vi "MPU_Stick_Write_General_Parameter.vi"(0 "ADCP in":refnum<class "ADCP.lvclass">, 5 "Parameter Name":string, 7 "Parameter Value":string, 11 "error out":errorcluster) -> (4 "ADCP out":refnum<class "ADCP.lvclass">, 15 "error out":errorcluster)   [LabVIEW 2017]
uses:
  Classes/ADCP.lvclass
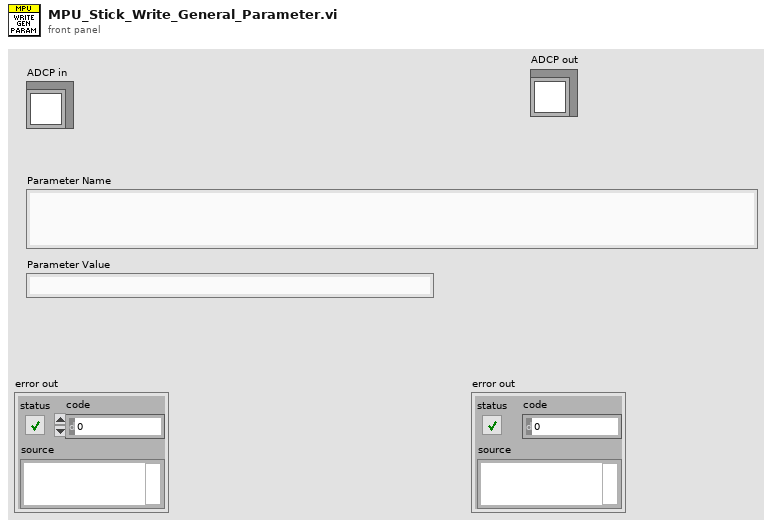
[diagram p1: front panel]
types:
  T1 = typedef "ADCP.lvclass/ADCP_Packet_Info.ctl" = cluster{"Priority":enum16{"LOW", "HIGH"}, "Type":enum16{"Data", "Connection Management", "Remote Request", "Error and status", "INVALID"}, "Node ID":i32, "Frame ID":i32, "Checksum valid ?":bool, "Current time (ms)":u32}
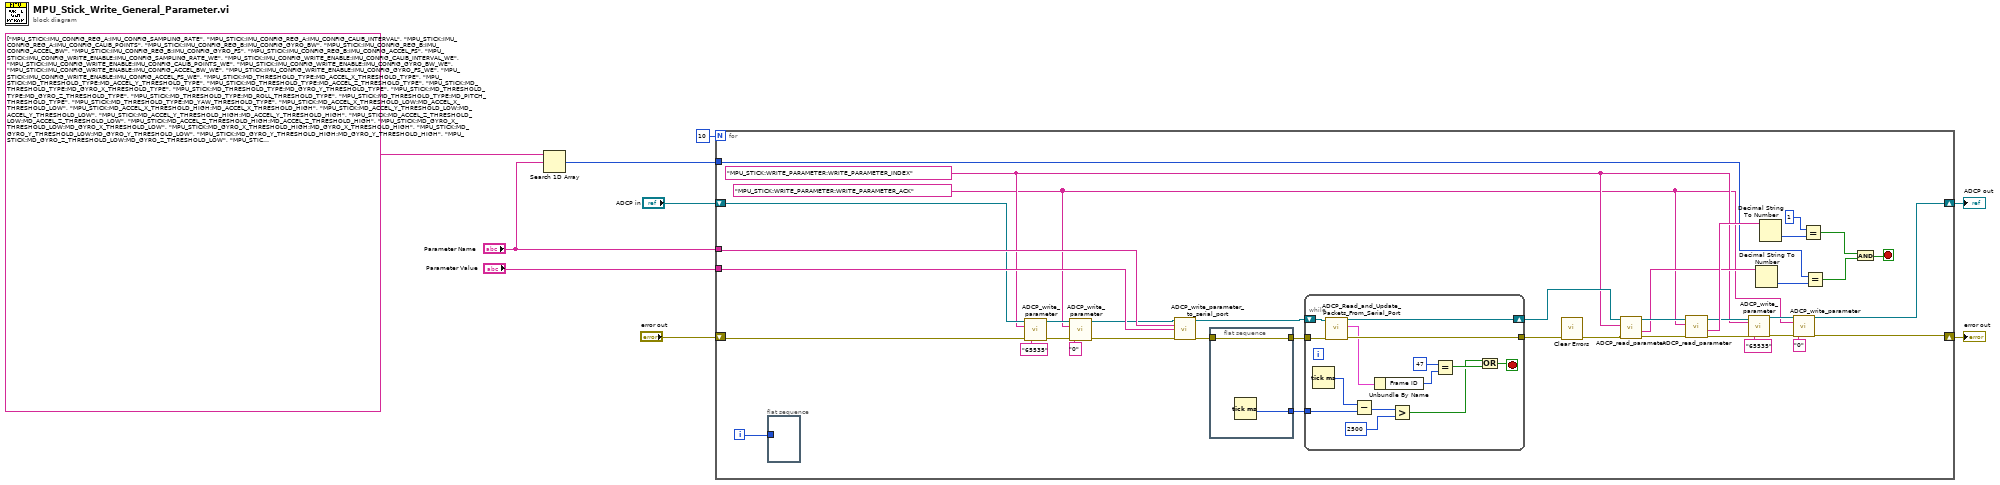
[diagram p0: block diagram]
diagram:
  n1 = Search 1D Array(1D array=string[] ["MPU_STICK:IMU_CONFIG_REG_A:IMU_CONFIG_SAMPLING_RATE", "MPU_STICK:IMU_CONFIG_REG_A:IMU_CONFIG_CALIB_INTERVAL", "MPU_STICK:IMU_CONFIG_REG_A:IMU_CONFIG_CALIB_POINTS", "MPU_STICK:IMU_CONFIG_REG_B:IMU_CONFIG_GYRO_BW", "MPU_STICK:IMU_CONFIG_REG_B:IMU_CONFIG_ACCEL_BW", "MPU_STICK:IMU_CONFIG_REG_B:IMU_CONFIG_GYRO_FS", "MPU_STICK:IMU_CONFIG_REG_B:IMU_CONFIG_ACCEL_FS", "MPU_STICK:IMU_CONFIG_WRITE_ENABLE:IMU_CONFIG_SAMPLING_RATE_WE", "MPU_STICK:IMU_CONFIG_WRITE_ENABLE:IMU_CONFIG_CALIB_INTERVAL_WE", "MPU_STICK:IMU_CONFIG_WRITE_ENABLE:IMU_CONFIG_CALIB_POINTS_WE", "MPU_STICK:IMU_CONFIG_WRITE_ENABLE:IMU_CONFIG_GYRO_BW_WE", "MPU_STICK:IMU_CONFIG_WRITE_ENABLE:IMU_CONFIG_ACCEL_BW_WE", "MPU_STICK:IMU_CONFIG_WRITE_ENABLE:IMU_CONFIG_GYRO_FS_WE", "MPU_STICK:IMU_CONFIG_WRITE_ENABLE:IMU_CONFIG_ACCEL_FS_WE", "MPU_STICK:MD_THRESHOLD_TYPE:MD_ACCEL_X_THRESHOLD_TYPE", "MPU_STICK:MD_THRESHOLD_TYPE:MD_ACCEL_Y_THRESHOLD_TYPE", "MPU_STICK:MD_THRESHOLD_TYPE:MD_ACCEL_Z_THRESHOLD_TYPE", "MPU_STICK:MD_THRESHOLD_TYPE:MD_GYRO_X_THRESHOLD_TYPE", "MPU_STICK:MD_THRESHOLD_TYPE:MD_GYRO_Y_THRESHOLD_TYPE", "MPU_STICK:MD_THRESHOLD_TYPE:MD_GYRO_Z_THRESHOLD_TYPE", "MPU_STICK:MD_THRESHOLD_TYPE:MD_ROLL_THRESHOLD_TYPE", "MPU_STICK:MD_THRESHOLD_TYPE:MD_PITCH_THRESHOLD_TYPE", "MPU_STICK:MD_THRESHOLD_TYPE:MD_YAW_THRESHOLD_TYPE", "MPU_STICK:MD_ACCEL_X_THRESHOLD_LOW:MD_ACCEL_X_THRESHOLD_LOW", "MPU_STICK:MD_ACCEL_X_THRESHOLD_HIGH:MD_ACCEL_X_THRESHOLD_HIGH", "MPU_STICK:MD_ACCEL_Y_THRESHOLD_LOW:MD_ACCEL_Y_THRESHOLD_LOW", "MPU_STICK:MD_ACCEL_Y_THRESHOLD_HIGH:MD_ACCEL_Y_THRESHOLD_HIGH", "MPU_STICK:MD_ACCEL_Z_THRESHOLD_LOW:MD_ACCEL_Z_THRESHOLD_LOW", "MPU_STICK:MD_ACCEL_Z_THRESHOLD_HIGH:MD_ACCEL_Z_THRESHOLD_HIGH", "MPU_STICK:MD_GYRO_X_THRESHOLD_LOW:MD_GYRO_X_THRESHOLD_LOW", "MPU_STICK:MD_GYRO_X_THRESHOLD_HIGH:MD_GYRO_X_THRESHOLD_HIGH", "MPU_STICK:MD_GYRO_Y_THRESHOLD_LOW:MD_GYRO_Y_THRESHOLD_LOW", "MPU_STICK:MD_GYRO_Y_THRESHOLD_HIGH:MD_GYRO_Y_THRESHOLD_HIGH", "MPU_STICK:MD_GYRO_Z_THRESHOLD_LOW:MD_GYRO_Z_THRESHOLD_LOW", "MPU_STICK:MD_GYRO_Z_THRESHOLD_HIGH:MD_GYRO_Z_THRESHOLD_HIGH", "MPU_STICK:MD_ROLL_THRESHOLD_LOW:MD_ROLL_THRESHOLD_LOW", "MPU_STICK:MD_ROLL_THRESHOLD_HIGH:MD_ROLL_THRESHOLD_HIGH", "MPU_STICK:MD_PITCH_THRESHOLD_LOW:MD_PITCH_THRESHOLD_LOW", "MPU_STICK:MD_PITCH_THRESHOLD_HIGH:MD_PITCH_THRESHOLD_HIGH", "MPU_STICK:MD_YAW_THRESHOLD_LOW:MD_YAW_THRESHOLD_LOW", "MPU_STICK:MD_YAW_THRESHOLD_HIGH:MD_YAW_THRESHOLD_HIGH", "MPU_STICK:MP_ROLL_FILTER_CONSTANT:MP_ROLL_FILTER_CONSTANT", "MPU_STICK:MP_PITCH_FILTER_CONSTANT:MP_PITCH_FILTER_CONSTANT", "MPU_STICK:MP_YAW_FILTER_CONSTANT:MP_YAW_FILTER_CONSTANT", "MPU_STICK:MD_WRITE_CONFIG:MD_ACCEL_X_THRESHOLD_LOW_WE", "MPU_STICK:MD_WRITE_CONFIG:MD_ACCEL_X_THRESHOLD_HIGH_WE", "MPU_STICK:MD_WRITE_CONFIG:MD_ACCEL_Y_THRESHOLD_LOW_WE", "MPU_STICK:MD_WRITE_CONFIG:MD_ACCEL_Y_THRESHOLD_HIGH_WE", "MPU_STICK:MD_WRITE_CONFIG:MD_ACCEL_Z_THRESHOLD_LOW_WE", "MPU_STICK:MD_WRITE_CONFIG:MD_ACCEL_Z_THRESHOLD_HIGH_WE", "MPU_STICK:MD_WRITE_CONFIG:MD_GYRO_X_THRESHOLD_LOW_WE", "MPU_STICK:MD_WRITE_CONFIG:MD_GYRO_X_THRESHOLD_HIGH_WE", "MPU_STICK:MD_WRITE_CONFIG:MD_GYRO_Y_THRESHOLD_LOW_WE", "MPU_STICK:MD_WRITE_CONFIG:MD_GYRO_Y_THRESHOLD_HIGH_WE", "MPU_STICK:MD_WRITE_CONFIG:MD_GYRO_Z_THRESHOLD_LOW_WE", "MPU_STICK:MD_WRITE_CONFIG:MD_GYRO_Z_THRESHOLD_HIGH_WE", "MPU_STICK:MD_WRITE_CONFIG:MD_ROLL_THRESHOLD_LOW_WE", "MPU_STICK:MD_WRITE_CONFIG:MD_ROLL_THRESHOLD_HIGH_WE", "MPU_STICK:MD_WRITE_CONFIG:MD_PITCH_THRESHOLD_LOW_WE", "MPU_STICK:MD_WRITE_CONFIG:MD_PITCH_THRESHOLD_HIGH_WE", "MPU_STICK:MD_WRITE_CONFIG:MD_YAW_THRESHOLD_LOW_WE", "MPU_STICK:MD_WRITE_CONFIG:MD_YAW_THRESHOLD_HIGH_WE", "MPU_STICK:MD_WRITE_CONFIG:MP_ROLL_FILTER_CONSTANT_WE", "MPU_STICK:MD_WRITE_CONFIG:MP_PITCH_FILTER_CONSTANT_WE", "MPU_STICK:MD_WRITE_CONFIG:MP_YAW_FILTER_CONSTANT_WE", "MPU_STICK:MD_WRITE_CONFIG:MD_ACCEL_X_THRESHOLD_TYPE_WE", "MPU_STICK:MD_WRITE_CONFIG:MD_ACCEL_Y_THRESHOLD_TYPE_WE", "MPU_STICK:MD_WRITE_CONFIG:MD_ACCEL_Z_THRESHOLD_TYPE_WE", "MPU_STICK:MD_WRITE_CONFIG:MD_GYRO_X_THRESHOLD_TYPE_WE", "MPU_STICK:MD_WRITE_CONFIG:MD_GYRO_Y_THRESHOLD_TYPE_WE", "MPU_STICK:MD_WRITE_CONFIG:MD_GYRO_Z_THRESHOLD_TYPE_WE", "MPU_STICK:MD_WRITE_CONFIG:MD_ROLL_THRESHOLD_TYPE_WE", "MPU_STICK:MD_WRITE_CONFIG:MD_PITCH_THRESHOLD_TYPE_WE", "MPU_STICK:MD_WRITE_CONFIG:MD_YAW_THRESHOLD_TYPE_WE", "MPU_STICK:LED_MODE_CONFIG:LED1_MODE", "MPU_STICK:LED_MODE_CONFIG:LED2_MODE", "MPU_STICK:LED_MODE_CONFIG:LED3_MODE", "MPU_STICK:LED_MODE_CONFIG:LED1_MODE_WE", "MPU_STICK:LED_MODE_CONFIG:LED2_MODE_WE", "MPU_STICK:LED_MODE_CONFIG:LED3_MODE_WE", "MPU_STICK:LED_UC_WRITE:LED1_UC_STATE", "MPU_STICK:LED_UC_WRITE:LED2_UC_STATE", "MPU_STICK:LED_UC_WRITE:LED3_UC_STATE", "MPU_STICK:LED_UC_WRITE:LED1_UC_DUTY", "MPU_STICK:LED_UC_WRITE:LED2_UC_DUTY", "MPU_STICK:LED_UC_WRITE:LED3_UC_DUTY", "MPU_STICK:LED_UC_WRITE:LED_UC_STATE_WE", "MPU_STICK:LED_UC_WRITE:LED_UC_DUTY_WE", "MPU_STICK:CONTROL:CONFIG_SAVE", "MPU_STICK:CONTROL:IMU_CALIBRATE", "MPU_STICK:CONTROL:MP_RESET", "MPU_STICK:CONTROL:CONFIG_SAVE_ACK", "MPU_STICK:CONTROL:IMU_CALIBRATE_ACK", "MPU_STICK:CONTROL:MP_RESET_ACK", "MPU_STICK:UPDATE_NODE_DATA:FRAME_ID", "MPU_STICK:WRITE_PARAMETER:WRITE_PARAMETER_INDEX", "MPU_STICK:WRITE_PARAMETER:WRITE_PARAMETER_ACK"] ("Write parameters"), element="Parameter Name") -> (index of element=w4:i32)  [unwired: 1 in]
  n2 = for {
    N: 10 -> [_]
    shift-right: [w18] -> w3
    shift-left: "ADCP in" -> [w44]
    tunnel: "Parameter Name" -> [w47]
    tunnel: "Parameter Value" -> [w48]
    shift-right: [w19] -> w2
    shift-left: "error out" -> [w45]
    tunnel: w4 -> [w28]
    i -> [w14]
    stop <- w17 stop-if-true
    w15 = "MPU_STICK:WRITE_PARAMETER:WRITE_PARAMETER_ACK" ("Parameter Name")
    w16 = "MPU_STICK:WRITE_PARAMETER:WRITE_PARAMETER_INDEX" ("Parameter Name")
    n3 = flat-sequence {
      tunnel: w14 -> [_]
      frame #0 {
      }
    }
    n4 = call "ADCP_write_parameter.vi"("ADCP in"=w44, "Parameter Name"=w16, "Parameter Value"="65535", "error in (no error)"=w45) -> ("ADCP out"=w42:refnum<class "ADCP.lvclass">, "error out"=w41:errorcluster)  [unwired: 9 in, 1 out]
    n5 = call "ADCP_write_parameter.vi"("ADCP in"=w42, "Parameter Name"=w15, "Parameter Value"="0", "error in (no error)"=w41) -> ("ADCP out"=w38:refnum<class "ADCP.lvclass">, "error out"=w39:errorcluster)  [unwired: 9 in, 1 out]
    n6 = call "ADCP_write_parameter_to_serial_port.vi"("ADCP In"=w38, "Parameter name"=w47, "Parameter value"=w48, "error in (no error)"=w39) -> ("ADCP out"=w46:refnum<class "ADCP.lvclass">, "error out"=w12:errorcluster)  [unwired: 8 in, 2 out]
    n7 = flat-sequence {
      tunnel: w12 -> [w50]
      tunnel: [w50] -> w11
      tunnel: [w49] -> w10
      frame #0 {
        n8 = Tick Count (ms)() -> (millisecond timer value=w49:u32)
      }
    }
    n9 = while {
      shift-right: [w63] -> w36
      shift-left: w46 -> [w64]
      tunnel: [w62] -> w13
      tunnel: w11 -> [w54]
      tunnel: w10 -> [w55]
      stop <- w61 stop-if-true
      n10 = Tick Count (ms)() -> (millisecond timer value=w56:u32)
      n11 = call "ADCP_Read_and_Update_Packets_From_Serial_Port.vi"("error in (no error)"=w54, "ADCP In"=w64) -> ("error out"=w62:errorcluster, "Packet Info"=w60:T1, "ADCP out"=w63:refnum<class "ADCP.lvclass">)  [unwired: 6 in, 1 out]
      n12 = Subtract(x=w56, y=w55) -> (x-y=w53:u32)
      n13 = Unbundle By Name(w60) -> ("Frame ID"=w59:i32)
      n14 = Greater?(x=w53, y=u32 2500) -> (0:w51:bool)
      n15 = Equal?(x=47, y=w59) -> (x = y?=w57:bool)
      n16 = Or(x=w51, y=w57) -> (x .or. y?=w61:bool)
    }
    n17 = call <vilib>:"Clear Errors.vi"("error in (no error)"=w13) -> ("error out"=w37:errorcluster)  [unwired: 5 in, 1 out]
    n18 = call "ADCP_read_parameter.vi"("error in (no error)"=w37, "Parameter Name"=w16, "ADCP In"=w36) -> ("error out"=w34:errorcluster, "Parameter Value"=w32:string, "ADCP out"=w35:refnum<class "ADCP.lvclass">)  [unwired: 5 in, 1 out]
    n19 = call "ADCP_read_parameter.vi"("error in (no error)"=w34, "Parameter Name"=w15, "ADCP In"=w35) -> ("error out"=w21:errorcluster, "Parameter Value"=w33:string, "ADCP out"=w20:refnum<class "ADCP.lvclass">)  [unwired: 5 in, 1 out]
    n20 = call "ADCP_write_parameter.vi"("ADCP in"=w20, "Parameter Name"=w16, "Parameter Value"="65535", "error in (no error)"=w21) -> ("ADCP out"=w24:refnum<class "ADCP.lvclass">, "error out"=w23:errorcluster)  [unwired: 9 in, 1 out]
    n21 = Decimal String To Number(string=w32) -> (number=w29:i32)  [unwired: 2 in, 1 out]
    n22 = Decimal String To Number(string=w33) -> (number=w31:i32)  [unwired: 2 in, 1 out]
    n23 = call "ADCP_write_parameter.vi"("ADCP in"=w24, "Parameter Name"=w15, "Parameter Value"="0", "error in (no error)"=w23) -> ("ADCP out"=w18:refnum<class "ADCP.lvclass">, "error out"=w19:errorcluster)  [unwired: 9 in, 1 out]
    n24 = Equal?(x=1, y=w31) -> (x = y?=w27:bool)
    n25 = Equal?(x=w28, y=w29) -> (x = y?=w26:bool)
    n26 = And(x=w27, y=w26) -> (x .and. y?=w17:bool)
  }
  "ADCP out" <- w3
  "error out" <- w2
